vi "HiSlope.vi"(1 "board":u32) -> ()   [LabVIEW 2017]
uses:
  ESLSCDLL.dll
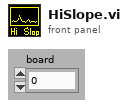
[diagram p1: front panel]
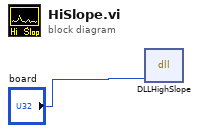
[diagram p0: block diagram]
diagram:
  n1 = dll-call lib="C:/ENTW/PCIE/64bit/lv64/lv64/board.vis/ESLSCDLL.dll" fn="DLLHighSlope"("drv"="board") -> ()  [unwired: 5 in, 2 out]
